vi "Linear Fit (multiple).vi"(8 "error in (no error)":errorcluster, 10 "Type":enum16{"y vs x", "x vs y"}(ring), 11 "XY-data":cluster{"X-array":dbl[], "Y-array":dbl[]}[](array[cluster]) {"Y-array" format="%.2p"; "X-array" format="%.2p"}) -> (0 "error out":errorcluster, 2 "Best Fits":cluster{"X-array":dbl[], "Y-array":dbl[]}[](array[cluster]), 3 "XY-data out":cluster{"X-array":dbl[], "Y-array":dbl[]}[](array[cluster]) {"Y-array" format="%.2p"; "X-array" format="%.2p"}, 4 "slopes":dbl[](array[numeric]), 5 "Lower Bounds":cluster{"X-array":dbl[], "Y-array":dbl[]}[](array[cluster]), 6 "intercepts":dbl[](array[numeric]), 7 "Upper Bounds":cluster{"X-array":dbl[], "Y-array":dbl[]}[](array[cluster]))   [LabVIEW 2016, in "xy_utilities.lvlib"]
doc: "Performs a linear fit using linear LS algorithm.\n\nWire data to the data input to determine the polymorphic instance to use or manually select the instance."
uses:
  xy_utilities.lvlib
  Swap X and Y.vi
  Swap X and Y (single).vi
  <vilib>/Analysis/6fits.llb/Linear Fit Intervals.vi
  <vilib>/Analysis/6fits.llb/Confidence Interval (Linear).vi
  <vilib>/Utility/error.llb/Error Cluster From Error Code.vi
  <vilib>/Analysis/6fits.llb/Linear Fit.vi
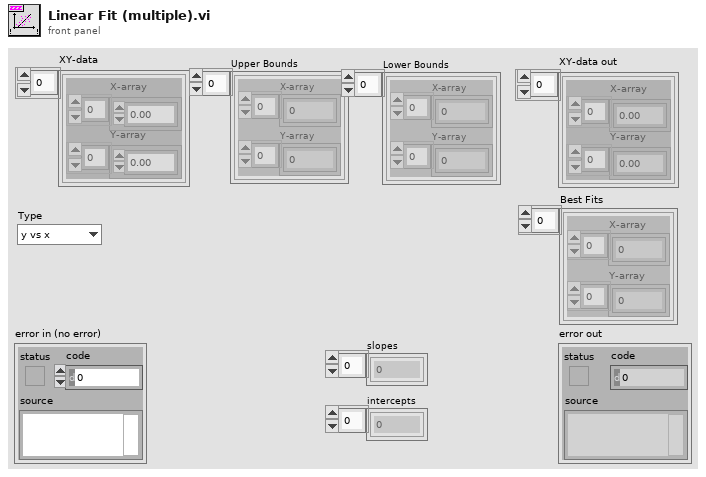
[diagram p1: front panel]
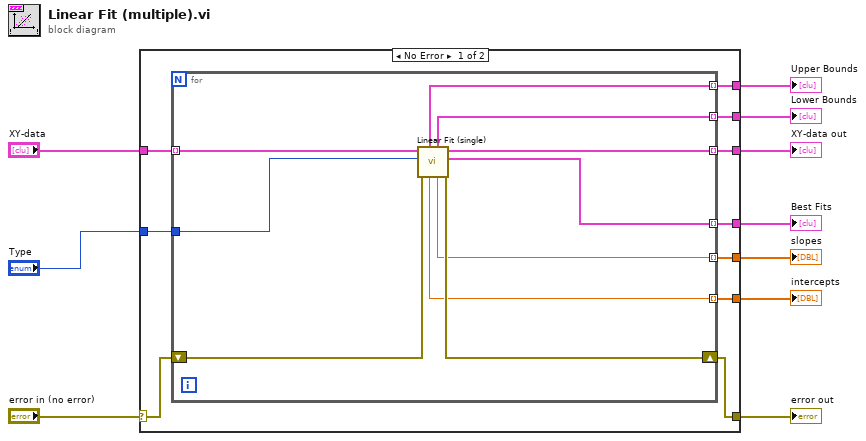
[diagram p0: block diagram]
diagram:
  n1 = case shown="No Error" "error in (no error)" {
    selector: "error in (no error)" -> [w18 w32]
    tunnel: [w17 w32] -> w9
    tunnel: "XY-data" -> [w20 w31]
    tunnel: [w19 w31] -> w7
    tunnel: "Type" -> [w16 _]
    tunnel: [w15 _] -> w5
    tunnel: [w14 _] -> w4
    tunnel: [w13 _] -> w3
    tunnel: [w12 _] -> w1
    tunnel: [w11 _] -> w2
    frame No Error {
      n2 = for {
        tunnel: w20 -> [w30] mode=indexing
        tunnel: [w25] -> w19 mode=indexing
        shift-right: [w27] -> w17
        shift-left: w18 -> [w28]
        tunnel: w16 -> [w29]
        tunnel: [w26] -> w15 mode=indexing
        tunnel: [w23] -> w14 mode=indexing
        tunnel: [w24] -> w13 mode=indexing
        tunnel: [w22] -> w12 mode=indexing
        tunnel: [w21] -> w11 mode=indexing
        n3 = call "Linear Fit (single).vi"("error in (no error)"=w28, "Type"=w29, "XY-data"=w30) -> ("error out"=w27:errorcluster, "Best Fit"=w26:cluster{"X-array":dbl[], "Y-array":dbl[]}, "XY-data out"=w25:cluster{"X-array":dbl[], "Y-array":dbl[]}, "slope"=w23:dbl, "Lower Bound"=w22:cluster{"X-array":dbl[], "Y-array":dbl[]}, "intercept"=w24:dbl, "Upper Bound"=w21:cluster{"X-array":dbl[], "Y-array":dbl[]})  [unwired: 2 in]
      }
    }
    frame Error {
    }
  }
  "error out" <- w9
  "XY-data out" <- w7
  "Best Fits" <- w5
  "slopes" <- w4
  "intercepts" <- w3
  "Upper Bounds" <- w2
  "Lower Bounds" <- w1
